vi "Periodic Tasks.vi"(8 "error in":errorcluster) -> ()   [LabVIEW 2017]
doc: "This VI runs in parallel to other tasks. It can contain as many user-defined periodic loops as you need. These can carry out PID or other sorts of timed response."
uses:
  <vilib>/Rock Robotics/WPI/DriverStation/WPI_DriverStationRobotMode2.ctl
  <vilib>/Rock Robotics/Network Tables/NT Read Boolean.vi
  Robot Global Data.vi
  Auto/AutoGlobals.vi
  SwerveRewrite/SwerveGlobals.vi
  <vilib>/Rock Robotics/Network Tables/NT Write Number.vi
  navx-mxp/labview/navX Library v2/navX Library v2.lvlib
panel:
  in  "EncoderRateConversion":dbl
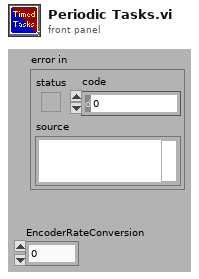
[diagram p1: front panel]
types:
  T1 = typedef "navX Library v2.lvlib/Z900_navX_DeviceTypeDef.ctl" = cluster{"Interface":cluster{"Protocol":T2, "Update Rate (4Hz-100Hz)":u8, "navX Open TypeDef":variant}, "Notify Packet":refnum<notifier>, "Loop VI Refnum":refnum<vi>, "Ready to Close Occurrence Refnum":refnum<k4>}
  T2 = typedef "navX Library v2.lvlib/Z900_navX_ProtocolTypeDef.ctl" = enum16{"SERIAL", "I2C", "SPI"}
  T3 = typedef "WPI_EncoderDevRef.ctl" = cluster{"DevStatus":errorcluster, "EncoderIndex":T4, "CounterIndex":T5, "DistancePerCount":dbl, "Decoding Type":T6}
  T4 = typedef "FPGA_EncoderIdx.ctl" = enum8{"Enc 0", "Enc 1", "Enc 2", "Enc 3", "Enc 4", "Enc 5", "Enc 6", "Enc 7", "Invalid"}
  T5 = typedef "FPGA_CounterCtrSystemIndex.ctl" = enum8{"Ctr 0", "Ctr 1", "Ctr 2", "Ctr 3", "Ctr 4", "Ctr 5", "Ctr 6", "Ctr 7", "Invalid"}
  T6 = typedef "WPI_EncoderType.ctl" = enum16{"1x", "2x", "4x"}
  T7 = typedef "WPI_DriverStationRobotMode2.ctl" = enum16{"Autonomous Disabled", "Autonomous Enabled", "Teleop Disabled", "Teleop Enabled", "Disconnected", "Finish", "Test Disabled", "Test Enabled", "Emergency Stopped"}
  T8 = cluster{"Yaw":dbl, "Roll":dbl, "Pitch":dbl, "Heading":dbl, "Fused Heading":dbl}
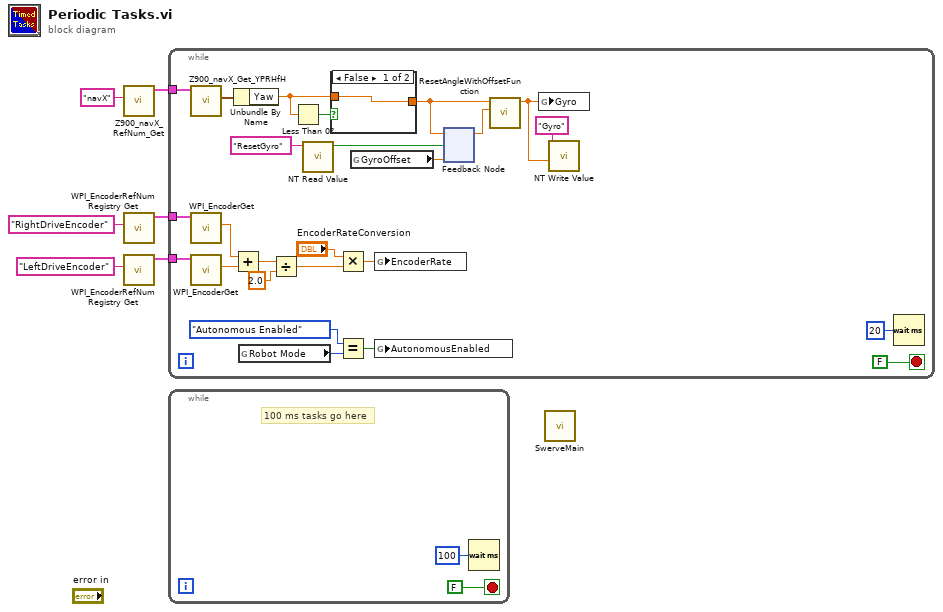
[diagram p0: block diagram]
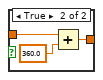
[diagram p2: hidden frame]
diagram:
  n1 = call "Z900_navX_RefNum_Get.vi"("refnum name"="navX") -> ("navX Device"=w5:T1)  [unwired: 9 in, 1 out]
  n2 = call <vilib>:"WPI_EncoderRefNum Registry Get.vi"("refnum name"="RightDriveEncoder") -> ("EncoderDevRef"=w2:T3)  [unwired: 9 in, 1 out]
  n3 = call <vilib>:"WPI_EncoderRefNum Registry Get.vi"("refnum name"="LeftDriveEncoder") -> ("EncoderDevRef"=w1:T3)  [unwired: 9 in, 1 out]
  n4 = while {
    tunnel: w5 -> [w14]
    tunnel: w2 -> [w23]
    tunnel: w1 -> [w22]
    stop <- FALSE stop-if-true
    n5 = call "Z900_navX_Get_YPRHfH.vi"("navX Device"=w14) -> ("YRPHfH"=w26:T8)  [unwired: 7 in, 3 out]
    n6 = call <vilib>:"WPI_EncoderGet.vi"("EncoderDevRef"=w23) -> ("Distance"=w19:dbl)  [unwired: 5 in, 5 out]
    n7 = call <vilib>:"WPI_EncoderGet.vi"("EncoderDevRef"=w22) -> ("Distance"=w18:dbl)  [unwired: 5 in, 5 out]
    n8 = Add(x=w19, y=w18) -> (x+y=w21:dbl)
    n9 = Unbundle By Name(w26) -> ("Yaw"=w24:dbl)
    n10 = global read "Robot Global Data.vi" "Robot Mode"() -> (w28:T7)
    n11 = Divide(x=w21, y=2.0) -> (x/y=w17:dbl)
    n12 = Less Than 0?(x=w24) -> (x < 0?=w25:bool)
    n13 = call-poly <vilib>:"NT Read Value.vi"("Name"="ResetGyro") -> ("Boolean"=w12:bool)  [unwired: 9 in, 1 out]
    n14 = case shown="False" w25 {
      tunnel: w24 -> [w32 w35]
      tunnel: [w32 w33] -> w9
      frame False {
      }
      frame True {
        n15 = Add(x=w35, y=360.0) -> (x+y=w33:dbl)
      }
    }
    n16 = Multiply(x="EncoderRateConversion", y=w17) -> (x*y=w16:dbl)
    n17 = Equal?(x=WPI_DriverStationRobotMode2."Autonomous Enabled" ("y"), y=w28) -> (x = y?=w29:bool)
    n18 = global read "SwerveGlobals.vi" "GyroOffset"() -> (w11:dbl)
    n19 = global write "AutoGlobals.vi" "EncoderRate"(w16) -> ()
    n20 = global write "AutoGlobals.vi" "AutonomousEnabled"(w29) -> ()
    n21 = feedback-in #1(w9, w12) -> ()
    n22 = feedback #1(w11) -> (w10:dbl)
    n23 = call "ResetAngleWithOffsetFunction.vi"("Offset"=w10, "AngleInput"=w9) -> ("AngleOutput"=w8:dbl)  [unwired: 9 in]
    n24 = global write "SwerveGlobals.vi" "Gyro"(w8) -> ()
    n25 = call-poly <vilib>:"NT Write Value.vi"("Numeric"=w8, "Name"="Gyro") -> ()  [unwired: 9 in, 1 out]
    n26 = Wait (ms)(milliseconds to wait=u32 20) -> ()  [unwired: 1 out]
  }
  n27 = while {
    stop <- FALSE stop-if-true
    # "100 ms tasks go here"
    n28 = Wait (ms)(milliseconds to wait=u32 100) -> ()  [unwired: 1 out]
  }
  n29 = call "SwerveMain.vi"() -> ()  [unwired: 12 in]
